vi "匹配一个或或者多个数字(指定开始数字).vi"() -> ()   [LabVIEW 2012]
uses:
  <vilib>/regexp/Match Regular Expression.xnode
panel:
  out "匹配后偏移量":i32=44
  out "匹配之后":string="."
  out "所有匹配":string="13804329998"
  out "匹配之前":string="My Phone Num is 021-87356659 and "
  in  "正则表达式":string="\\b1\\d+\\b"
  in  "字符串":string="My Phone Num is 021-87356659 and 13804329998."
  # "\\d+表示匹配一个或者更多连续数字"
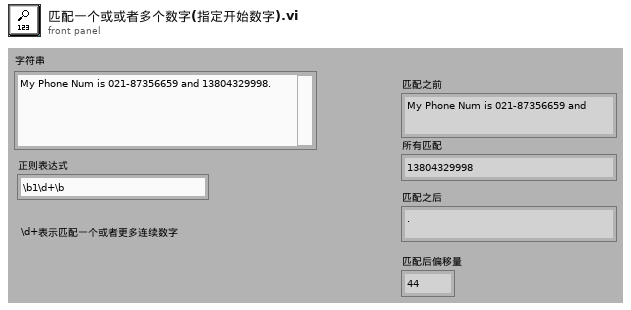
[diagram p1: front panel]
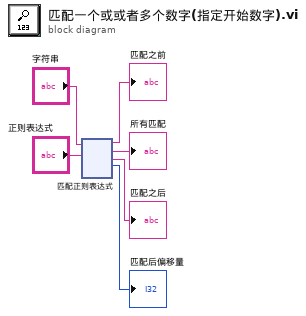
[diagram p0: block diagram]
diagram:
  n1 = xnode "匹配正则表达式"("输入字符串"="字符串", "正则表达式"="正则表达式") -> ("匹配之前"=→"匹配之前":string, "所有匹配"=→"所有匹配":string, "匹配之后"=→"匹配之后":string, "匹配后偏移量"=→"匹配后偏移量":i32)  [unwired: 4 in, 1 out]
